vi "PredetControlSequence (SubVI).vi"(1 "Predet Freq (Hz)":dbl=20.0 format="%#_13g", 2 "Stop Button":bool, 3 "Error In":errorcluster) -> (0 "PredetState":T1, 10 "Error Out":errorcluster)   [LabVIEW 2016]
uses:
  PredetControl.ctl
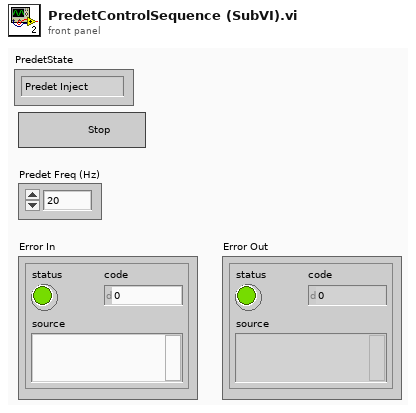
[diagram p1: front panel]
types:
  T1 = typedef "PredetControl.ctl" = enum16{"Predet Inject", "Predet Fire", "Stop"}
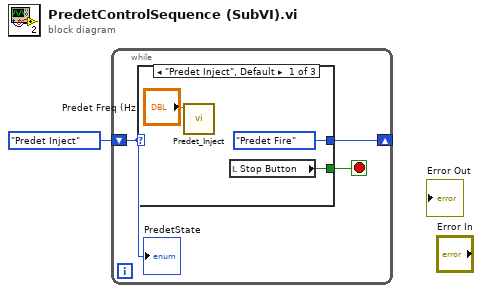
[diagram p0: block diagram]
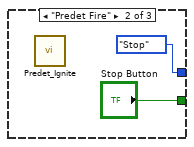
[diagram p2: hidden frame]
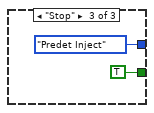
[diagram p3: hidden frame]
diagram:
  n1 = while {
    shift-right: [w3] -> _
    shift-left: PredetControl."Predet Inject" -> [w4]
    stop <- w2 stop-if-true
    n2 = case shown="\"Predet Inject\", Default" w4 {
      tunnel: [PredetControl."Predet Fire" PredetControl."Stop" PredetControl."Predet Inject"] -> w3
      tunnel: [w6 "Stop Button" TRUE] -> w2
      frame "Predet Inject", Default {
        n3 = call "Predet_Inject.vi"("Predet Freq (Hz)"="Predet Freq (Hz)") -> ()  [unwired: 11 in]
        n4 = local read "Stop Button"() -> (w6:bool)
      }
      frame "Predet Fire" {
        n5 = call "Predet_Ignite.vi"() -> ()  [unwired: 10 in, 2 out]
      }
      frame "Stop" {
      }
    }
    "PredetState" <- w4
  }
